vi "RF627.vi"() -> ()   [LabVIEW 2019]
doc: "This example VI calls the .NET DLL that accompanies it, which is a .NET class built in C# to emulate a very basic calculator."
uses:
  C:/Users/aagolovachev/Desktop/RLD_T14_2dScan/src/RF62X/RF62X-SDK/examples/LabVIEW/rf62Xsdk.dll
  rf62Xsdk.dll
panel:
  out "size(s)":i32
  out "Capacity":i32
  out "ReadParams":bool
  out "Connect":bool
  in  "DeviceIDX":i32
  in  "protocol":i32(ring)=1 items=["SERVICE_PROTOKOL"=1, "ETHERNET_IP"=2, "MODBUS_TCP"=3]
  out "N of Sensors":i32
  out "xemr":u16
  out "zmr":u16
  out "Disconnect":bool
  in  "?":bool
  out "N Points":i32
  out "XY Graph":cluster{"X":sgl, "Z":sgl}[](graph)
  out "SdkInit":bool
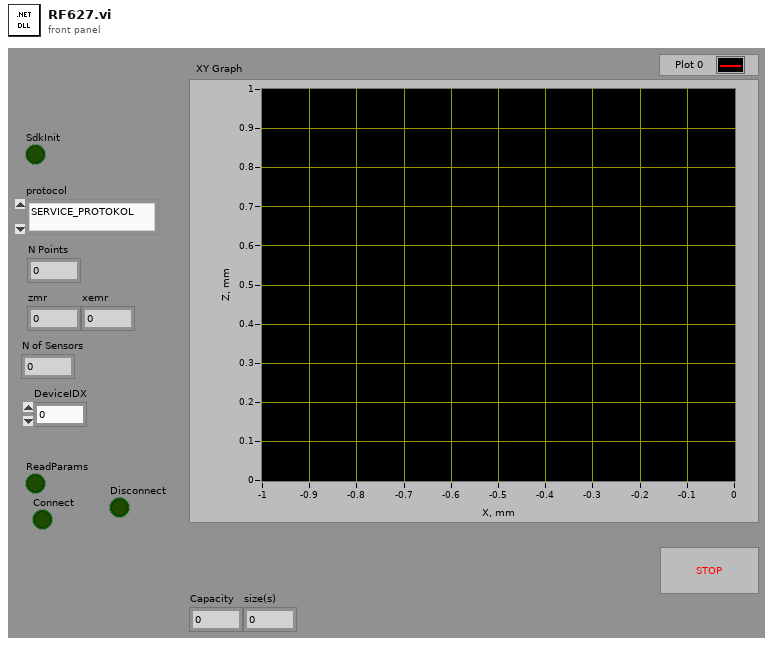
[diagram p1: front panel]
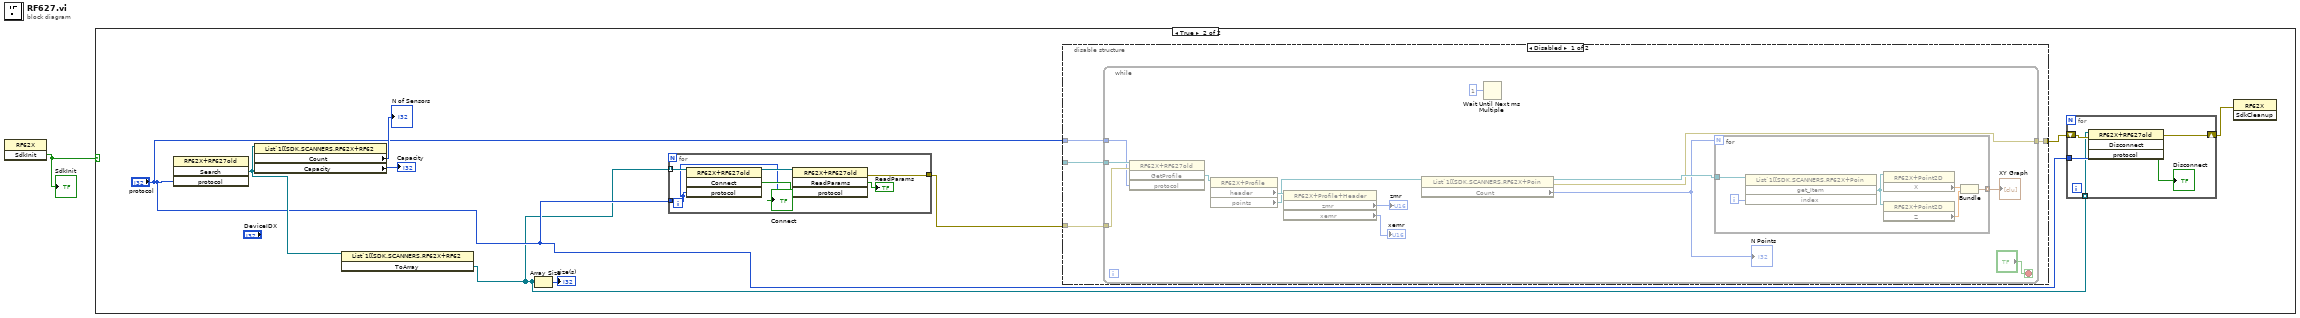
[diagram p0: block diagram]
diagram:
  n1 = invoke class="RF62X" method="SdkInit"() -> ("SdkInit"=w1:bool)  [unwired: 3 in, 2 out]
  "SdkInit" <- w1
  n2 = case shown="True" w1 {
    frame False {
    }
    frame True {
      n3 = invoke class="RF62X+RF627old" method="Search"("protocol"="protocol") -> ("Search"=w6:refnum<k24>)  [unwired: 3 in, 3 out]
      n4 = property class="List`1[[SDK.SCANNERS.RF62X+RF62"(reference=w6) -> ("Count"=→"N of Sensors":i32, "Capacity"=→"Capacity":i32)  [unwired: 1 in, 2 out]
      n5 = invoke class="List`1[[SDK.SCANNERS.RF62X+RF62" method="ToArray"(reference=w6) -> ("ToArray"=w2:refnum<k24>[])  [unwired: 2 in, 2 out]
      n6 = Array Size(array=w2) -> (size(s)=→"size(s)":i32)
      n7 = for {
        tunnel: w2 -> [w46] mode=indexing
        tunnel: "protocol" -> [w42]
        tunnel: [w43] -> w3
        n8 = invoke class="RF62X+RF627old" method="Connect"(reference=w46, "protocol"=w42) -> (reference out=w45:refnum<k24>, "Connect"=→"Connect":bool)  [unwired: 2 in, 2 out]
        n9 = invoke class="RF62X+RF627old" method="ReadParams"(reference=w45, "protocol"=w42) -> (error out=w43:errorcluster, "ReadParams"=→"ReadParams":bool)  [unwired: 2 in, 2 out]
      }
      n10 = disable-structure shown="Disabled" {
        disable-tunnel: [w19 w40] -> w8
        disable-tunnel: _ -> [w18 _]
        disable-tunnel: w3 -> [w17 w40]
        disable-tunnel: "protocol" -> [w16 _]
        frame Disabled {
          n11 = while {
            tunnel: [w30] -> w19
            tunnel: w18 -> [w23]
            tunnel: w17 -> [w22]
            tunnel: w16 -> [w21]
            stop <- "?" stop-if-true
            n12 = invoke class="RF62X+RF627old" method="GetProfile"(reference=w23, error in=w22, "protocol"=w21) -> ("GetProfile"=w27:refnum<k24>)  [unwired: 1 in, 3 out]
            n13 = property class="RF62X+Profile"(reference=w27) -> ("header"=w24:refnum<k24>, "points"=w20:refnum<k24>)  [unwired: 1 in, 2 out]
            n14 = property class="RF62X+Profile+Header"(reference=w24) -> ("zmr"=→"zmr":u16, "xemr"=→"xemr":u16)  [unwired: 1 in, 2 out]
            n15 = property class="List`1[[SDK.SCANNERS.RF62X+Poin"(reference=w20) -> (reference out=w31:refnum<k24>, error out=w30:errorcluster, "Count"=w29:i32)  [unwired: 1 in]
            "N Points" <- w29
            n16 = Wait Until Next ms Multiple(millisecond multiple=u32 1 ("millisecond timer value")) -> ()  [unwired: 1 out]
            n17 = for {
              N: w29 -> [_]
              tunnel: [w38] -> w32 mode=indexing
              tunnel: w31 -> [w34]
              i -> [w39]
              n18 = invoke class="List`1[[SDK.SCANNERS.RF62X+Poin" method="get_Item"(reference=w34, "index"=w39) -> ("get_Item"=w37:refnum<k24>)  [unwired: 2 in, 3 out]
              n19 = property class="RF62X+Point2D"(reference=w37) -> ("X"=w36:sgl)  [unwired: 1 in, 2 out]
              n20 = property class="RF62X+Point2D"(reference=w37) -> ("Z"=w35:sgl)  [unwired: 1 in, 2 out]
              n21 = Bundle("X"=w36, "Z"=w35) -> (w38:cluster{"X":sgl, "Z":sgl})  [unwired: 1 in]
            }
            "XY Graph" <- w32
          }
        }
        frame Enabled {
        }
      }
      n22 = for {
        tunnel: "protocol" -> [w12]
        shift-right: [w14] -> w9
        shift-left: w8 -> [w13]
        tunnel: w2 -> [w11] mode=indexing
        n23 = invoke class="RF62X+RF627old" method="Disconnect"(reference=w11, error in=w13, "protocol"=w12) -> (error out=w14:errorcluster, "Disconnect"=→"Disconnect":bool)  [unwired: 1 in, 2 out]
      }
      n24 = invoke class="RF62X" method="SdkCleanup"(error in=w9) -> ()  [unwired: 2 in, 3 out]
    }
  }
